vi "Measurement Logic.vi"() -> ()   [LabVIEW 2021, in "Ramp-Up Time_PMIC.lvlib"]
uses:
  Ramp-Up Time_PMIC.lvlib
  <vilib>/Plug-In SDKs/Measurements/Measure Call Context/Measure Call Context.lvclass
  Measurement Results.ctl
  Measurement Configuration.ctl
  <instrlib>/niDCPower/nidcpower.llb/niDCPower Source Mode.ctl
  <instrlib>/niDCPower/nidcpower.llb/niDCPower Wait For Event - Event.ctl
  <instrlib>/niScope/Controls/niScope trigger slope.ctl
  <instrlib>/niDCPower/nidcpower.llb/niDCPower Output Function.ctl
  <instrlib>/niDCPower/nidcpower.llb/niDCPower Aperture Time Units.ctl
  <instrlib>/niDCPower/nidcpower.llb/niDCPower Get Channel Name From String.vi
  <instrlib>/niScope/Utility/niScope Get Channel Name From String.vi
  <instrlib>/niScope/Configure/Trigger/niScope Configure Trigger Digital.vi
  <instrlib>/niDCPower/nidcpower.llb/niDCPower Configure Digital Edge Measure Trigger With Channels.vi
  <instrlib>/niDCPower/nidcpower.llb/niDCPower Configure Digital Edge Source Trigger With Channels.vi
  <instrlib>/niScope/Acquire/Fetch/niScope Fetch WDT.vi
panel:
  in  "measurement configuration":T1={"Source resource name"="", "Source current limit"=0.25, "Source sample rate"=1800000.0, "Source voltage set point 1(V1)"=7.0, "Source voltage set point 2(V2)"=20.0, "Source transient response"=1042, "Source voltage gain bandwidth"=2000.0, "Source voltage compensation frequency"=3530.0, "Source voltage pole-zero ratio"=2.0, "Source maximum power"=300.0, "Source voltage ramp rate"=6550.0, "Source voltatge V2 time"=0.005, "Source voltage V1 time"=0.005, "Load enable/disable"=TRUE, "Load resource name"="", "Load sense"=1009, "Load voltage limit range"=6.0, "Load current level"=1.0, "Scope enable/disable"=TRUE, "Scope resource name"="", "Scope output channel name"="0", "Scope sample rate"=1800000.0, "Scope probe attenuation"=1.0, "Scope vertical range"=10.0, "Scope vertical coupling"=enum."DC", "Load current level range"=4.0, "Load source delay"=1.0, "Source ramp start percentage(%)"=10.0, "Source ramp stop percentage(%)"=90.0, "Source sense"=1009} {"Source sense" items=["Local"=1008, "Remote"=1009]; "Scope vertical range" format="%.2f"; "Scope probe attenuation" format="%.1f"; "Scope sample rate" step=1000000.0 format="%#.2g"; "Load current level" format="%.1f"; "Load voltage limit range" step=1000000.0 format="%#.2g"; "Load sense" items=["Local"=1008, "Remote"=1009]; "Source voltage V1 time" format="%#_8g"; "Source transient response" items=["Slow"=1041, "Normal"=1038, "Fast"=1039, "Custom"=1042]}
  out "measurement results":T2
  out "measure call context out":refnum<class "Measure Call Context.lvclass">
  in  "measure call context in":refnum<class "Measure Call Context.lvclass">
  out "error out":errorcluster
  in  "error in":errorcluster
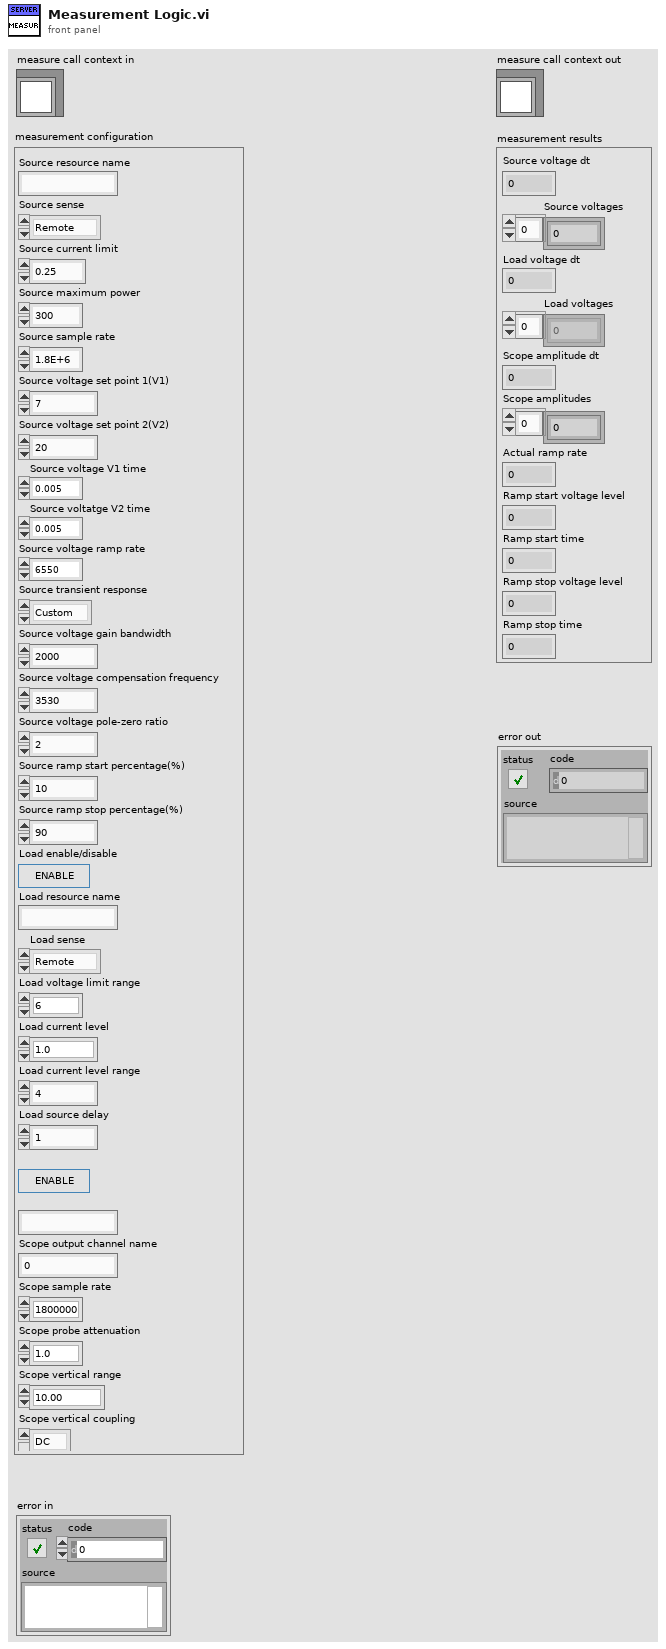
[diagram p1: front panel]
types:
  T1 = typedef "Ramp-Up Time_PMIC.lvlib/Measurement Configuration.ctl" = cluster{"Source resource name":string, "Source current limit":dbl, "Source sample rate":dbl, "Source voltage set point 1(V1)":dbl, "Source voltage set point 2(V2)":dbl, "Source transient response":i32, "Source voltage gain bandwidth":dbl, "Source voltage compensation frequency":dbl, "Source voltage pole-zero ratio":dbl, "Source maximum power":dbl, "Source voltage ramp rate":dbl, "Source voltatge V2 time":dbl, "Source voltage V1 time":dbl, "Load enable/disable":bool, "Load resource name":string, "Load sense":i32, "Load voltage limit range":dbl, "Load current level":dbl, "Scope enable/disable":bool, "Scope resource name":string, "Scope output channel name":string, "Scope sample rate":dbl, "Scope probe attenuation":dbl, "Scope vertical range":dbl, "Scope vertical coupling":enum32{"AC", "DC"}, "Load current level range":dbl, "Load source delay":dbl, "Source ramp start percentage(%)":dbl, "Source ramp stop percentage(%)":dbl, "Source sense":i32}
  T2 = typedef "Ramp-Up Time_PMIC.lvlib/Measurement Results.ctl" = cluster{"Source voltage dt":dbl, "Source voltages":dbl[], "Load voltage dt":dbl, "Load voltages":dbl[], "Scope amplitude dt":dbl, "Scope amplitudes":dbl[], "Actual ramp rate":dbl, "Ramp start voltage level":dbl, "Ramp start time":dbl, "Ramp stop voltage level":dbl, "Ramp stop time":dbl}
  T3 = cluster{"Source out":refnum<k15>, "Source channel name":string, "Load out":refnum<k15>, "Load channel name":string, "Scope out":refnum<k15>, "Scope channel name":string, "Source terminal name":string, "Start source terminal name":string, "Measure load and scope terminal name":string, "Measure record length smu":i32, "Aperture time":dbl, "Measure record length scope":i32, "measurement results":T2}
  T4 = typedef "niDCPower Wait For Event - Event.ctl" = i32
  T5 = typedef "niDCPower Source Mode.ctl" = i32
  T6 = typedef "niScope trigger slope.ctl" = i32
  T7 = typedef "niDCPower Aperture Time Units.ctl" = i32
  T8 = typedef "niDCPower Output Function.ctl" = i32
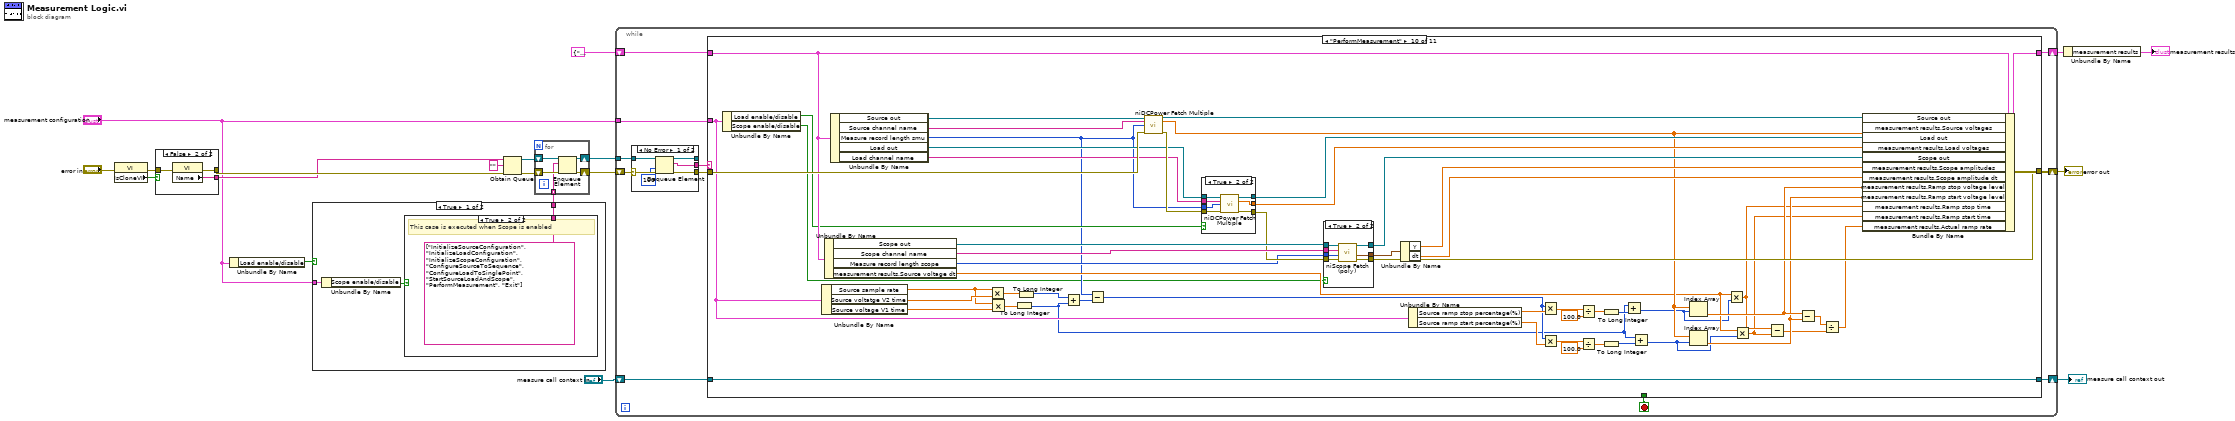
[diagram p0: block diagram]
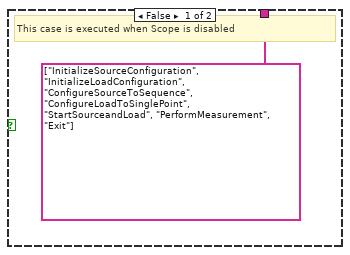
[diagram p2: hidden frame]
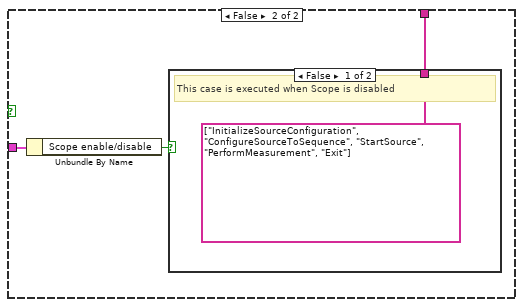
[diagram p3: hidden frame]
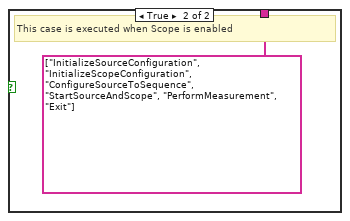
[diagram p4: hidden frame]
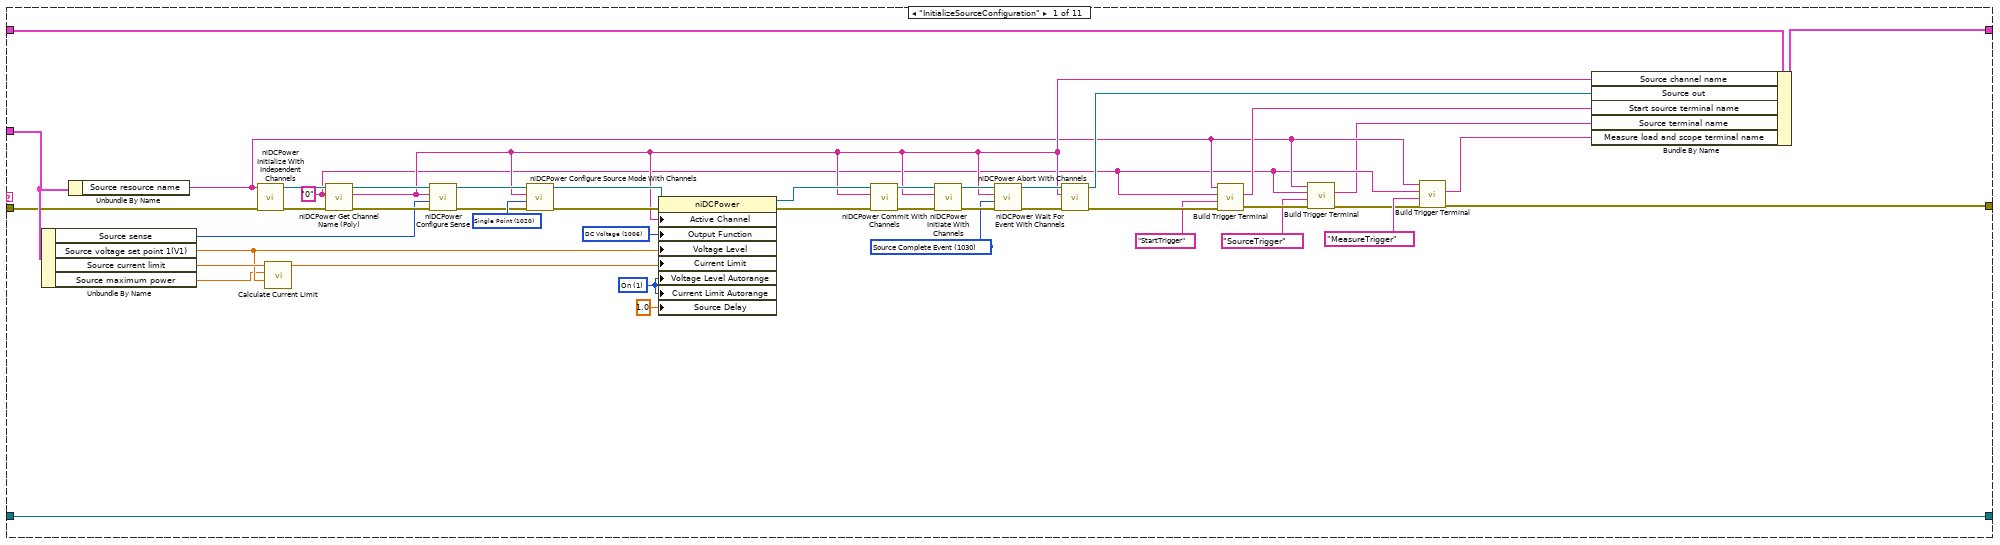
[diagram p5: hidden frame]
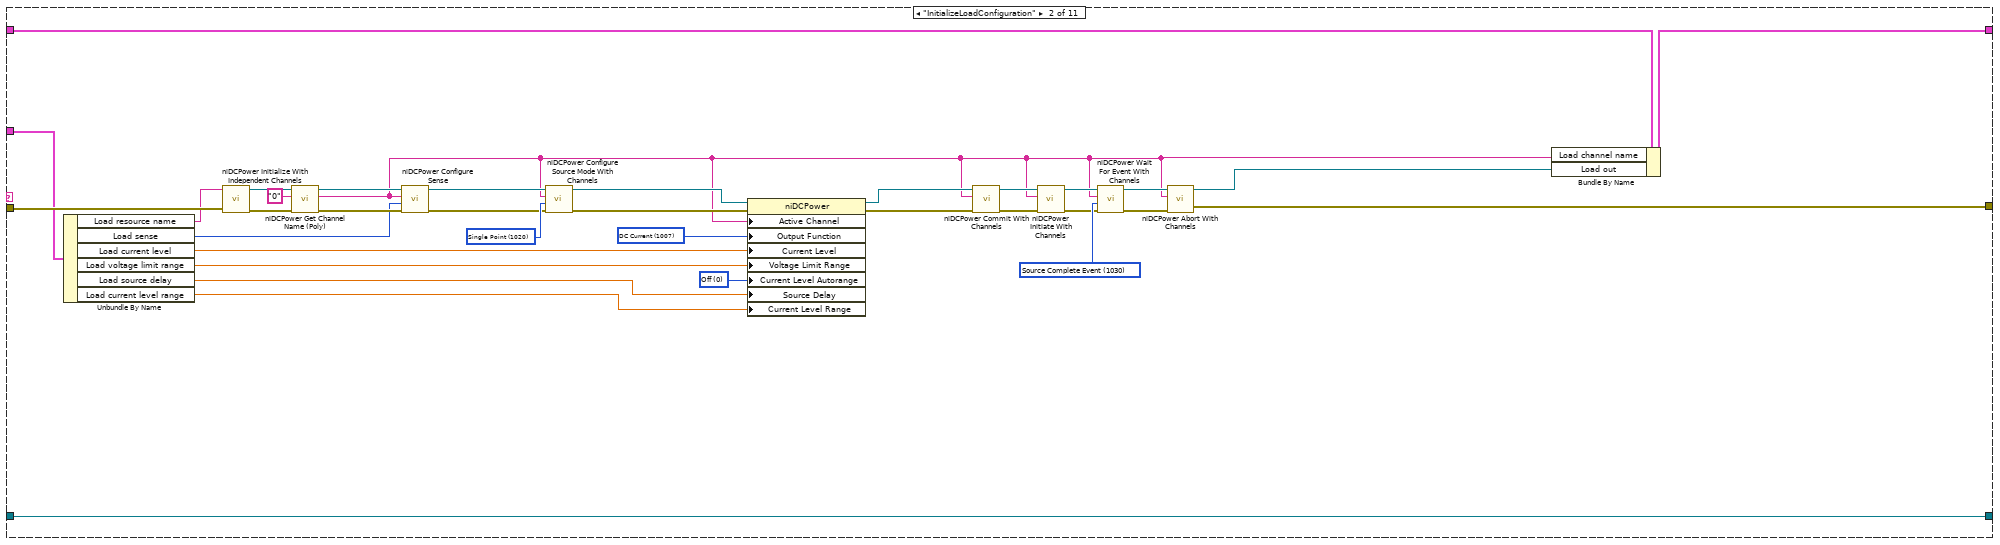
[diagram p6: hidden frame]
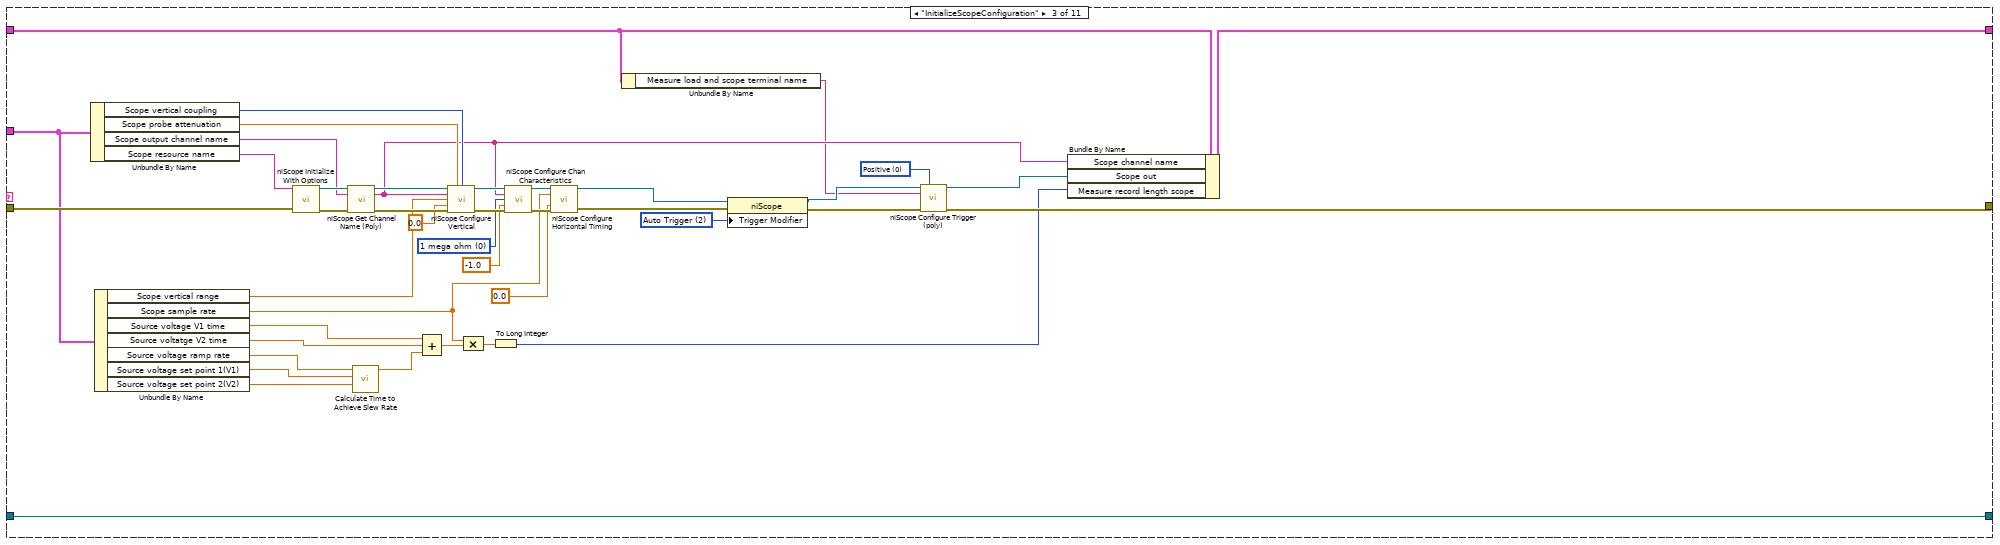
[diagram p7: hidden frame]
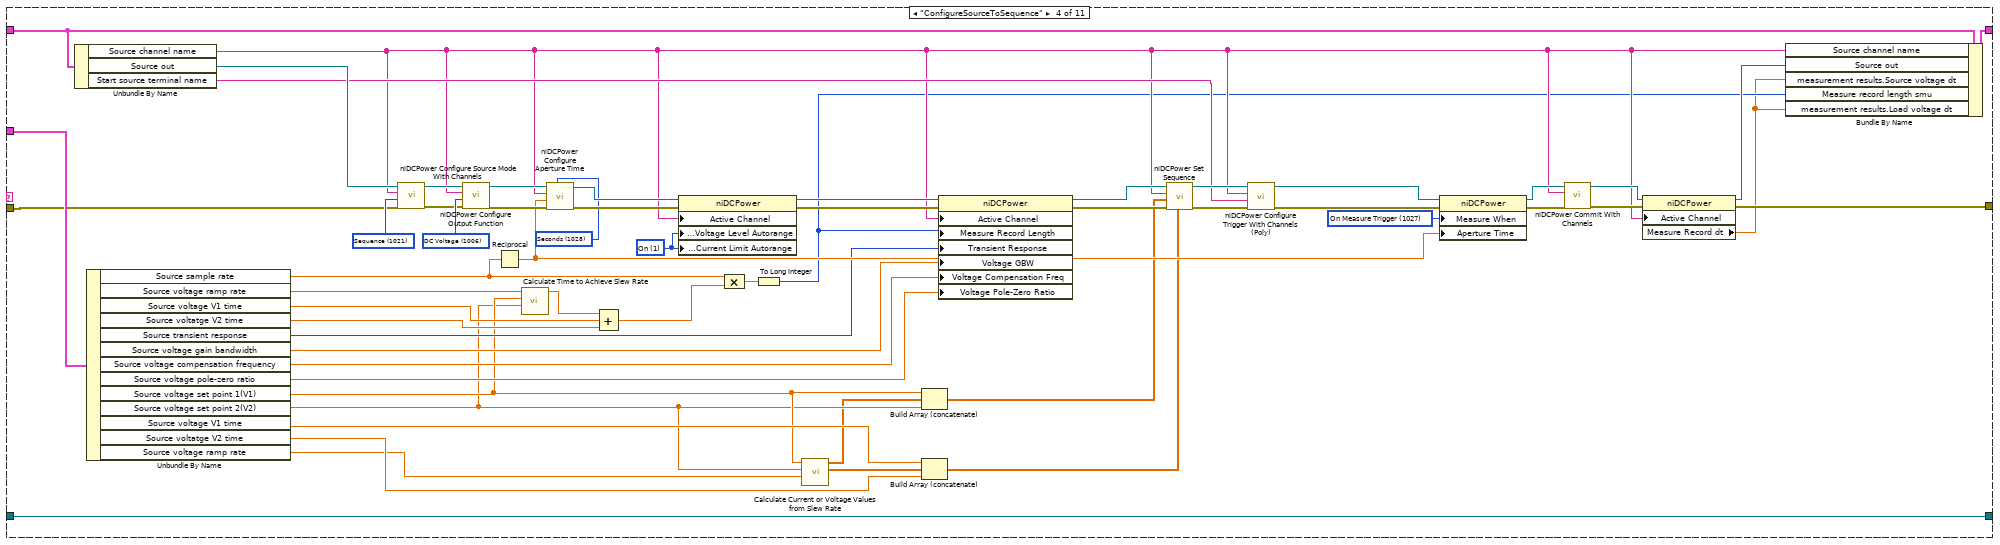
[diagram p8: hidden frame]
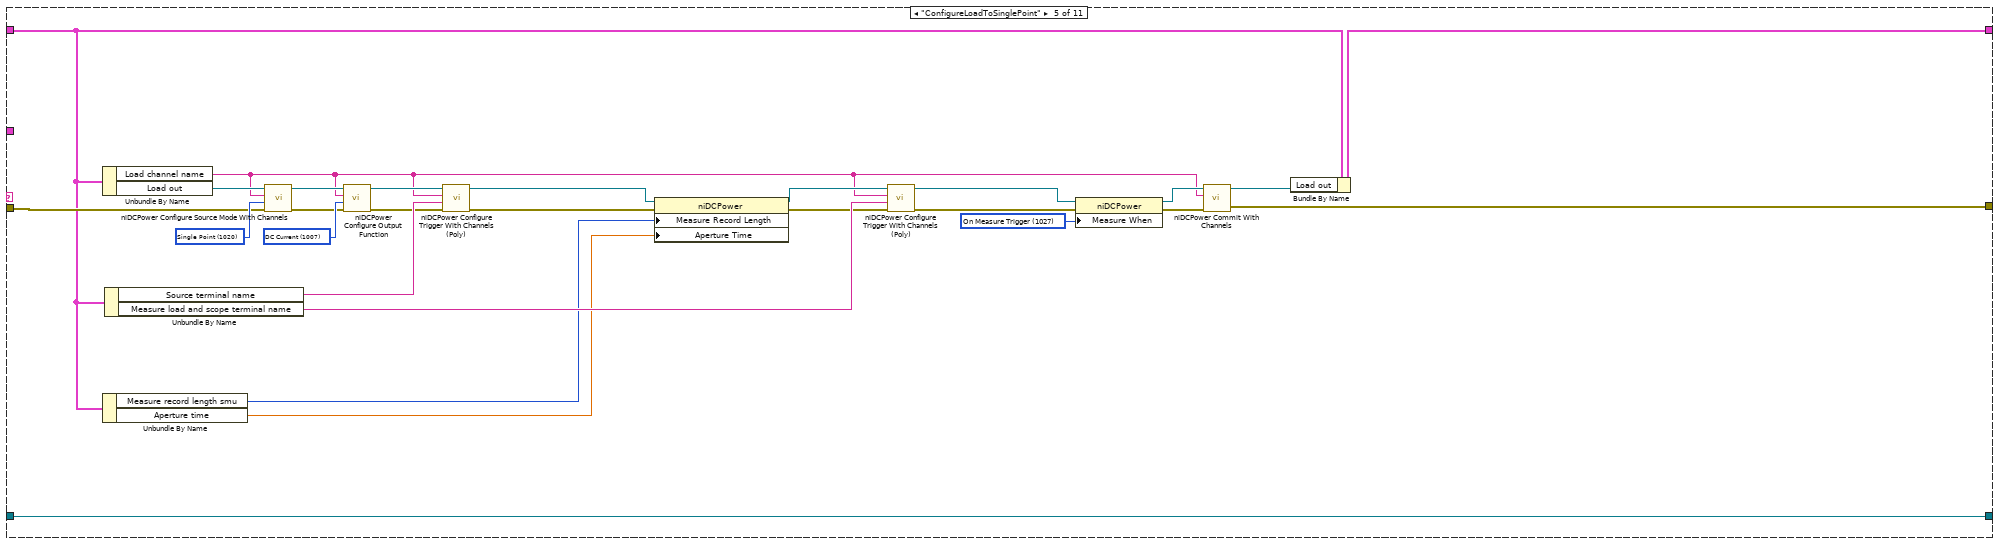
[diagram p9: hidden frame]
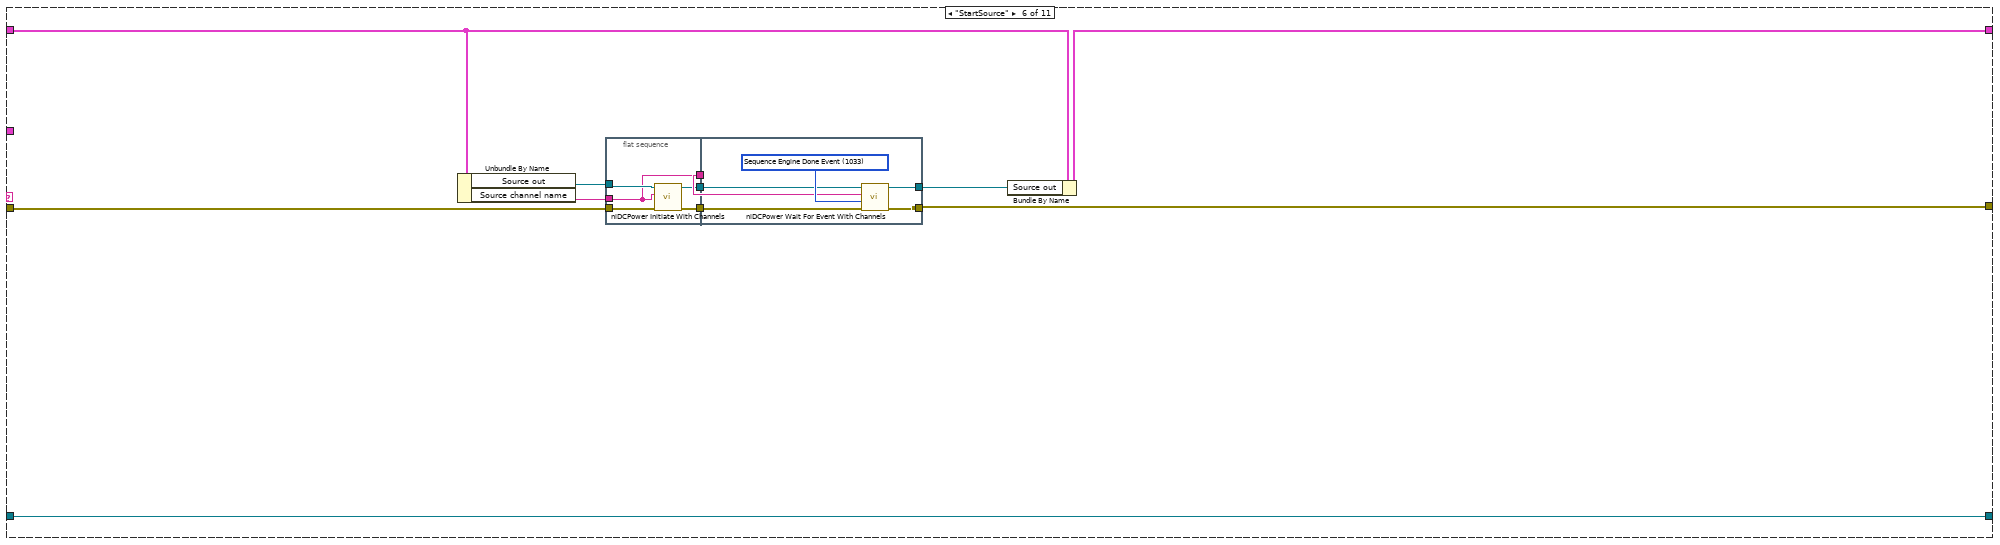
[diagram p10: hidden frame]
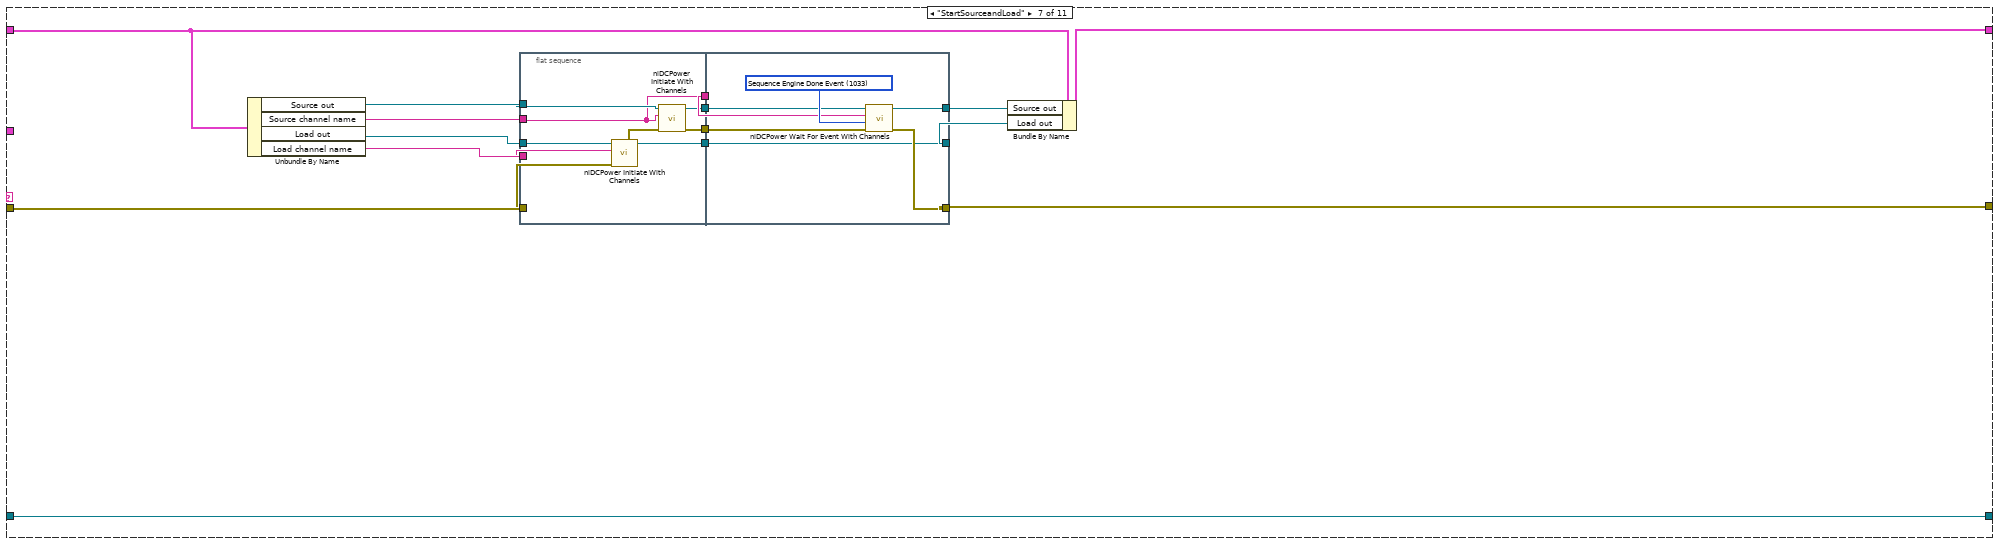
[diagram p11: hidden frame]
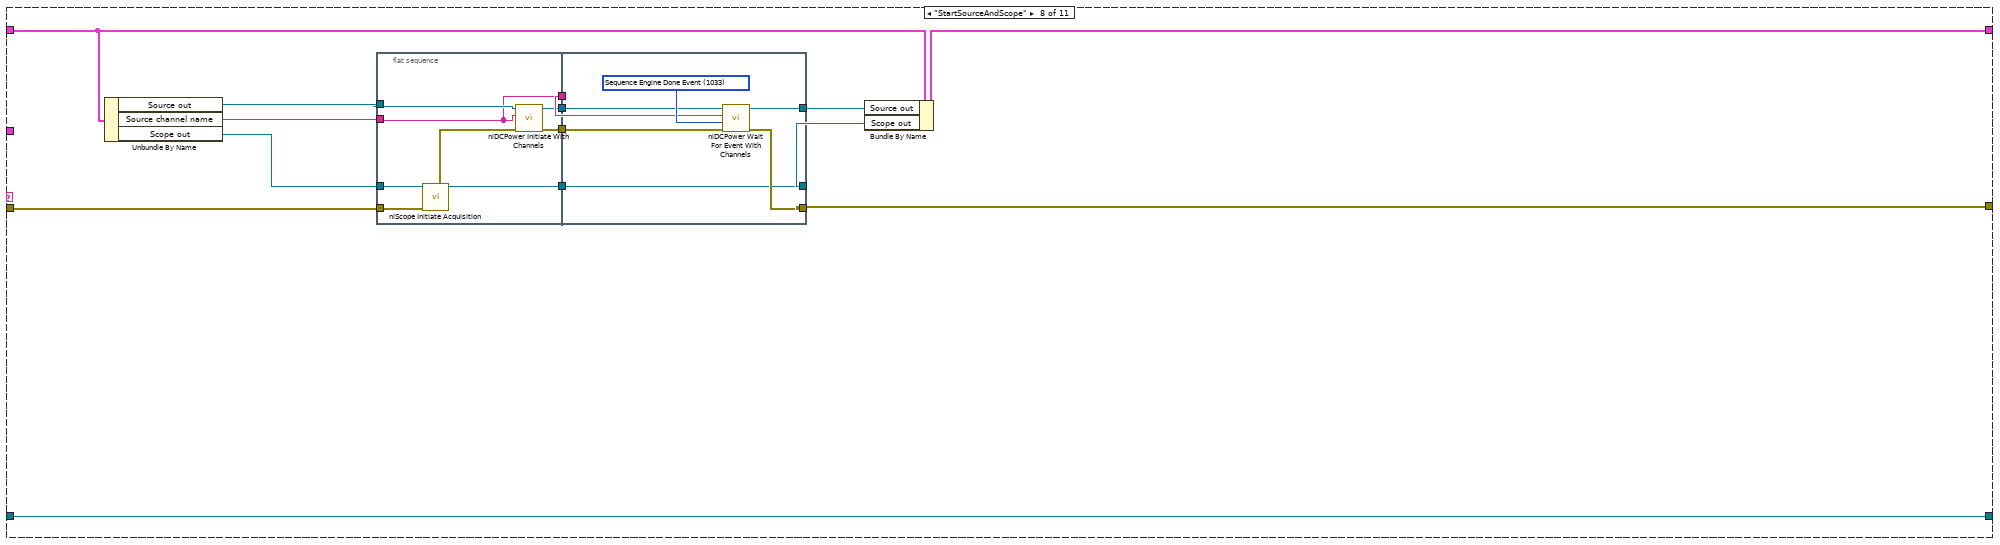
[diagram p12: hidden frame]
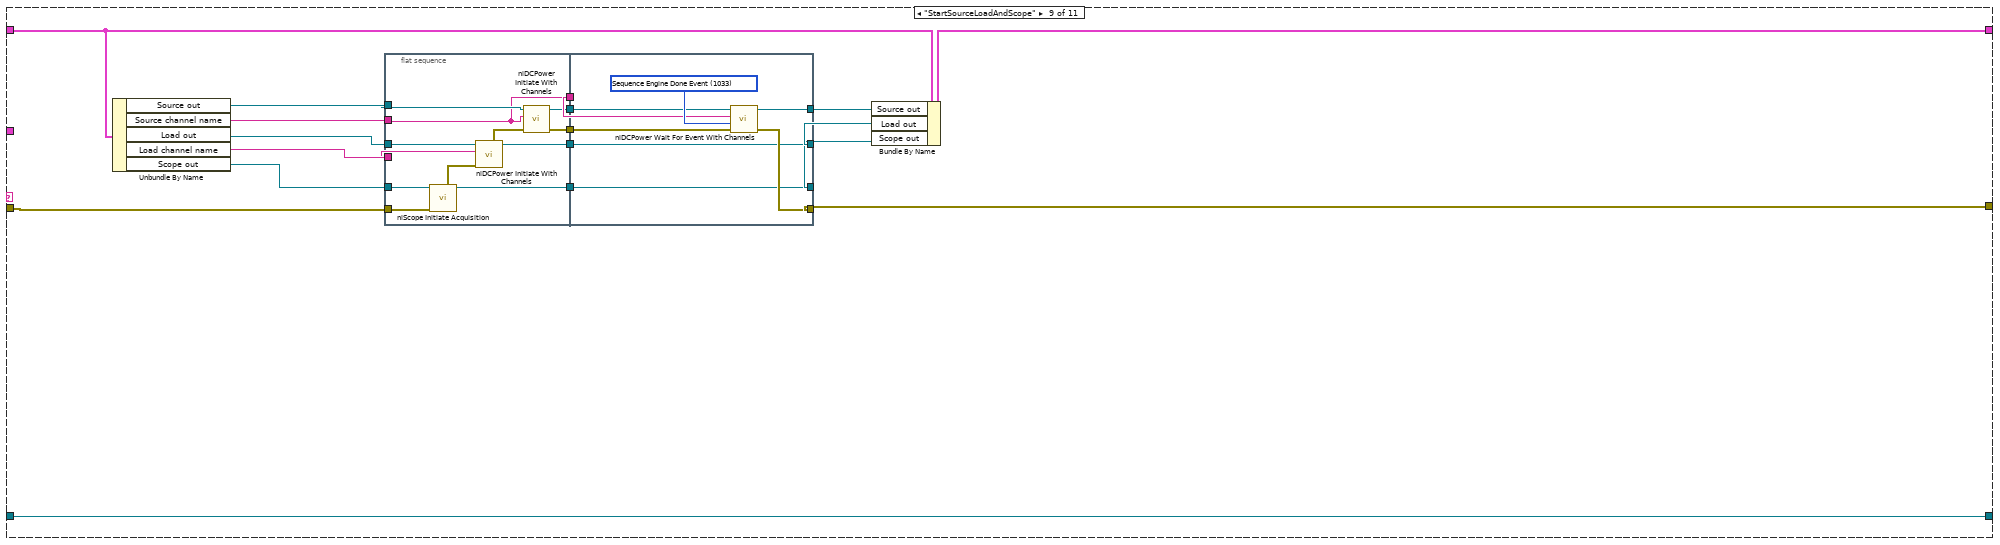
[diagram p13: hidden frame]
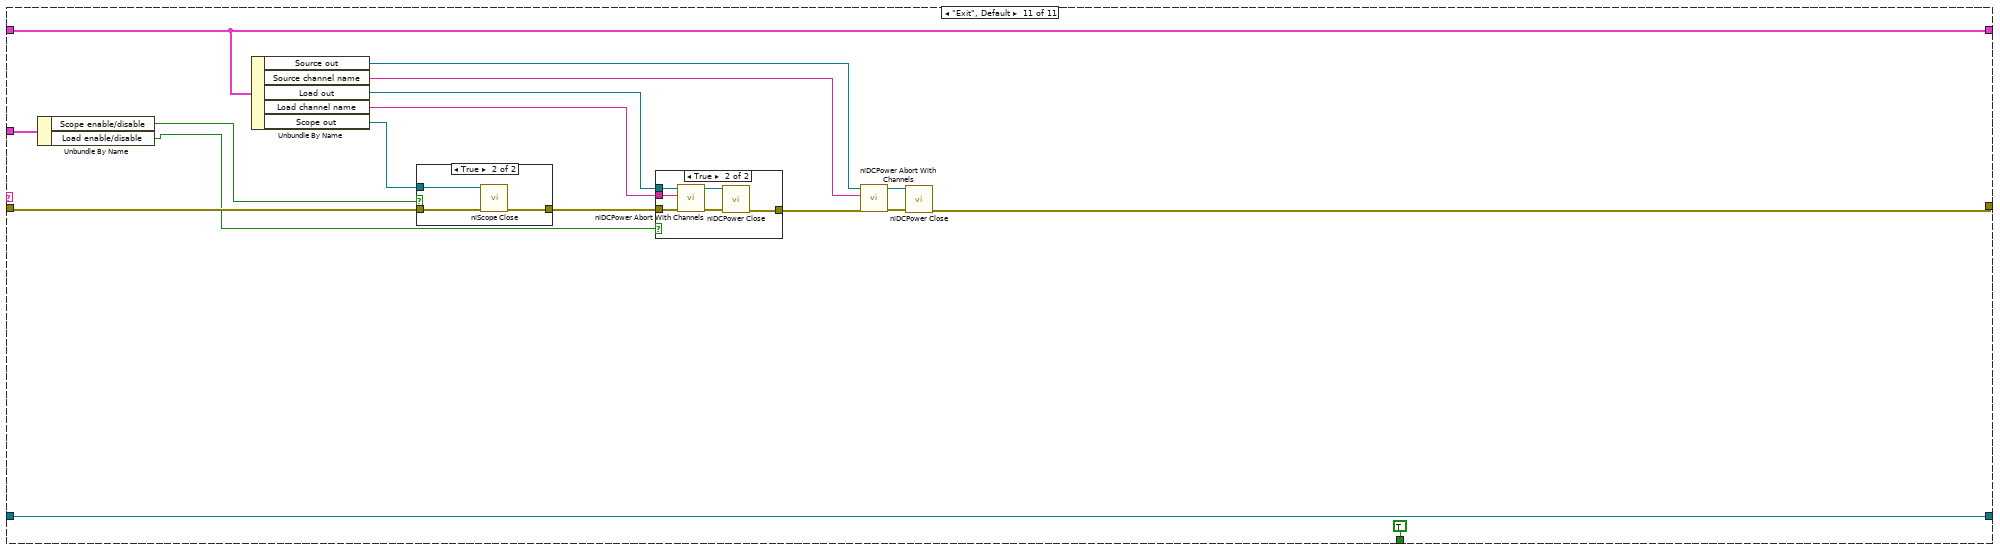
[diagram p16: hidden frame]
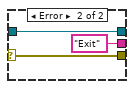
[diagram p19: hidden frame]
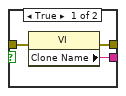
[diagram p20: hidden frame]
diagram:
  n1 = property class="VI"(error in="error in") -> (error out=w18:errorcluster, "IsCloneVI"=w19:bool)  [unwired: 1 in, 1 out]
  n2 = case shown="False" w19 {
    tunnel: [w22 w25] -> w17
    tunnel: [w21 w24] -> w16
    tunnel: w18 -> [w20 w23]
    frame True {
      n3 = property class="VI"(error in=w20) -> (error out=w22:errorcluster, "Clone Name"=w21:string)  [unwired: 1 in, 1 out]
    }
    frame False {
      n4 = property class="VI"(error in=w23) -> (error out=w25:errorcluster, "Name"=w24:string)  [unwired: 1 in, 1 out]
    }
  }
  n5 = Unbundle By Name("measurement configuration") -> ("Load enable/disable"=w3:bool)
  n6 = case shown="True" w3 {
    tunnel: [w26 w33] -> w12
    tunnel: "measurement configuration" -> [w27 w31]
    frame True {
      n7 = Unbundle By Name(w27) -> ("Scope enable/disable"=w28:bool)
      n8 = case shown="True" w28 {
        tunnel: [string[] ["InitializeSourceConfiguration", "InitializeLoadConfiguration", "ConfigureSourceToSequence", "ConfigureLoadToSinglePoint", "StartSourceandLoad", "PerformMeasurement", "Exit"] ("Step sequence") string[] ["InitializeSourceConfiguration", "InitializeLoadConfiguration", "InitializeScopeConfiguration", "ConfigureSourceToSequence", "ConfigureLoadToSinglePoint", "StartSourceLoadAndScope", "PerformMeasurement", "Exit"] ("Step sequence")] -> w26
        frame False {
          # "This case is executed when Scope is disabled"
        }
        frame True {
          # "This case is executed when Scope is enabled"
        }
      }
    }
    frame False {
      n9 = Unbundle By Name(w31) -> ("Scope enable/disable"=w32:bool)
      n10 = case shown="False" w32 {
        tunnel: [string[] ["InitializeSourceConfiguration", "ConfigureSourceToSequence", "StartSource", "PerformMeasurement", "Exit"] ("Step sequence") string[] ["InitializeSourceConfiguration", "InitializeScopeConfiguration", "ConfigureSourceToSequence", "StartSourceAndScope", "PerformMeasurement", "Exit"] ("Step sequence")] -> w33
        frame False {
          # "This case is executed when Scope is disabled"
        }
        frame True {
          # "This case is executed when Scope is enabled"
        }
      }
    }
  }
  n11 = Obtain Queue(name (unnamed)=w16, element data type="", error in (no error)=w17) -> (queue out=w14:refnum<queue>, error out=w15:errorcluster)  [unwired: 2 in, 1 out]
  n12 = for {
    shift-right: [w38] -> w11
    shift-left: w14 -> [w40]
    shift-right: [w37] -> w10
    shift-left: w15 -> [w39]
    tunnel: w12 -> [w36] mode=indexing
    n13 = Enqueue Element(queue=w40, element=w36, error in (no error)=w39) -> (queue out=w38:refnum<queue>, error out=w37:errorcluster)  [unwired: 1 in, 1 out]
  }
  n14 = while {
    tunnel: w11 -> [w51]
    shift-right: [w44] -> w8
    shift-left: w10 -> [w50]
    tunnel: "measurement configuration" -> [w48]
    shift-right: [w46] -> w6
    shift-left: T3 {"Source out"="", "Source channel name"="", "Load out"="", "Load channel name"="", "Scope out"="", "Scope channel name"="", "Source terminal name"="", "Start source terminal name"="", "Measure load and scope terminal name"="", "Measure record length smu"=0, "Aperture time"=0.0, "Measure record length scope"=0, "measurement results"={"Source voltage dt"=0.0, "Source voltages"=[0.0], "Load voltage dt"=0.0, "Load voltages"=[], "Scope amplitude dt"=0.0, "Scope amplitudes"=[0.0], "Actual ramp rate"=0.0, "Ramp start voltage level"=0.0, "Ramp start time"=0.0, "Ramp stop voltage level"=0.0, "Ramp stop time"=0.0}} -> [w47]
    shift-right: [w42] -> w1
    shift-left: "measure call context in" -> [w41]
    stop <- w43 stop-if-true
    n15 = case shown="No Error" w50 {
      selector: w50 -> [w481 w485]
      tunnel: w51 -> [w483 w484]
      tunnel: [w482 "Exit" ("t")] -> w49
      tunnel: [w480 w485] -> w45
      tunnel: [w478 w484] -> _
      frame No Error {
        n16 = Dequeue Element(queue=w483, timeout in ms (-1)=100, error in (no error)=w481) -> (queue out=w478:refnum<queue>, element=w482:string, error out=w480:errorcluster)  [unwired: 1 out]
      }
      frame Error {
      }
    }
    n17 = case shown="\"PerformMeasurement\"" w49 {
      tunnel: w48 -> [w74 w102 w143 w195 _ _ _ _ _ w392 w462]
      tunnel: w47 -> [w73 w99 w140 w194 w232 w261 w281 w317 w341 w430 w463]
      tunnel: [w72 w100 w173 w229 w231 w260 w280 w312 w340 w429 w463] -> w46
      tunnel: w45 -> [w71 w103 w144 w192 w233 w262 w282 w316 w342 w431 w466]
      tunnel: [w57 w101 w138 w183 w230 w259 w279 w313 w339 w428 w465] -> w44
      tunnel: [_ _ _ _ _ _ _ _ _ _ TRUE] -> w43
      tunnel: [w69 w131 w137 w188 w256 w258 w293 w311 w356 w421 w456] -> w42
      tunnel: w41 -> [w69 w131 w137 w188 w256 w258 w293 w311 w356 w421 w456]
      frame "InitializeSourceConfiguration" {
        w55 = "0" ("index")
        w80 = 1 items=["Off", "On"] ("Source:DC Voltage:Voltage Level Autorange")
        w81 = T4 1030 items=["Source Complete Event"=1030, "Measure Complete Event"=1031, "Sequence Iteration Complete Event"=1032, "Sequence Engine Done Event"=1033, "Pulse Complete Event"=1051, "Ready For Pulse Trigger Event"=1052] ("event")
        w92 = T5 1020 items=["Single Point"=1020, "Sequence"=1021] ("source mode")
        w87 = 1006 items=["DC Voltage"=1006, "DC Current"=1007, "Pulse Voltage"=1049, "Pulse Current"=1050] ("Source:Output Function")
        n18 = Unbundle By Name(w74) -> ("Source sense"=w52:i32, "Source voltage set point 1(V1)"=w67:dbl, "Source current limit"=w68:dbl, "Source maximum power"=w66:dbl)
        n19 = Unbundle By Name(w74) -> ("Source resource name"=w56:string)
        n20 = call <instrlib>:"niDCPower Initialize With Independent Channels.vi"("error in (no error)"=w71, "resource name"=w56) -> ("error out"=w78:errorcluster, "instrument handle out"=w82:refnum<k15>)  [unwired: 8 in]
        n21 = call "Calculate Current Limit.vi"("Voltage value"=w67, "Maximum power"=w66, "Current limit in"=w68) -> ("Current limit out"=w65:dbl)  [unwired: 8 in]
        n22 = call-poly <instrlib>:"niDCPower Get Channel Name (Poly).vi"("error in (no error)"=w78, "index"=w55, "instrument handle"=w82) -> ("error out"=w77:errorcluster, "name"=w76:string, "instrument handle out"=w79:refnum<k15>)  [unwired: 6 in]
        n23 = call <instrlib>:"niDCPower Configure Sense.vi"("error in (no error)"=w77, "sense"=w52, "channel name"=w76, "instrument handle"=w79) -> ("error out"=w90:errorcluster, "instrument handle out"=w88:refnum<k15>)  [unwired: 6 in]
        n24 = call <instrlib>:"niDCPower Configure Source Mode With Channels.vi"("error in (no error)"=w90, "source mode"=w92, "channel name"=w76, "instrument handle"=w88) -> ("error out"=w91:errorcluster, "instrument handle out"=w89:refnum<k15>)  [unwired: 6 in]
        n25 = property class="niDCPower"(reference=w89, error in=w91, "Active Channel"=w76, "Output Function"=w87, "Voltage Level"=w67, "Current Limit"=w65, "Voltage Level Autorange"=w80, "Current Limit Autorange"=w80, "Source Delay"=1.0 ("Source:Advanced:Source Delay")) -> (reference out=w93:refnum<k15>, error out=w94:errorcluster)
        n26 = call <instrlib>:"niDCPower Commit With Channels.vi"("error in (no error)"=w94, "channel name"=w76, "instrument handle"=w93) -> ("error out"=w96:errorcluster, "instrument handle out"=w95:refnum<k15>)  [unwired: 7 in]
        n27 = call <instrlib>:"niDCPower Initiate With Channels.vi"("error in (no error)"=w96, "channel name"=w76, "instrument handle"=w95) -> ("error out"=w83:errorcluster, "instrument handle out"=w84:refnum<k15>)  [unwired: 7 in]
        n28 = call <instrlib>:"niDCPower Wait For Event With Channels.vi"("error in (no error)"=w83, "event"=w81, "channel name"=w76, "instrument handle"=w84) -> ("error out"=w86:errorcluster, "instrument handle out"=w85:refnum<k15>)  [unwired: 6 in]
        n29 = call <instrlib>:"niDCPower Abort With Channels.vi"("error in (no error)"=w86, "channel name"=w76, "instrument handle"=w85) -> ("error out"=w64:errorcluster, "instrument handle out"=w75:refnum<k15>)  [unwired: 7 in]
        n30 = call "Build Trigger Terminal.vi"("error in (no error)"=w64, "Trigger/Event Name"="StartTrigger", "Channel Name"=w55, "Resource Name"=w56) -> ("error out"=w62:errorcluster, "Terminal Name"=w60:string)  [unwired: 6 in]
        n31 = call "Build Trigger Terminal.vi"("error in (no error)"=w62, "Trigger/Event Name"="SourceTrigger", "Channel Name"=w55, "Resource Name"=w56) -> ("error out"=w58:errorcluster, "Terminal Name"=w53:string)  [unwired: 6 in]
        n32 = call "Build Trigger Terminal.vi"("error in (no error)"=w58, "Trigger/Event Name"="MeasureTrigger", "Channel Name"=w55, "Resource Name"=w56) -> ("error out"=w57:errorcluster, "Terminal Name"=w54:string)  [unwired: 6 in]
        n33 = Bundle By Name(cluster=w73, "Source channel name"=w76, "Source out"=w75, "Start source terminal name"=w60, "Source terminal name"=w53, "Measure load and scope terminal name"=w54) -> (w72:T3)
      }
      frame "InitializeLoadConfiguration" {
        w126 = T5 1020 items=["Single Point"=1020, "Sequence"=1021] ("source mode")
        w119 = T4 1030 items=["Source Complete Event"=1030, "Measure Complete Event"=1031, "Sequence Iteration Complete Event"=1032, "Sequence Engine Done Event"=1033, "Pulse Complete Event"=1051, "Ready For Pulse Trigger Event"=1052] ("event")
        w114 = 0 items=["Off", "On"] ("Source:DC Current:Current Level Autorange")
        w115 = 1007 items=["DC Voltage"=1006, "DC Current"=1007, "Pulse Voltage"=1049, "Pulse Current"=1050] ("Source:Output Function")
        n34 = Unbundle By Name(w102) -> ("Load resource name"=w98:string, "Load sense"=w97:i32, "Load current level"=w108:dbl, "Load voltage limit range"=w107:dbl, "Load source delay"=w113:dbl, "Load current level range"=w106:dbl)
        n35 = call <instrlib>:"niDCPower Initialize With Independent Channels.vi"("error in (no error)"=w103, "resource name"=w98) -> ("error out"=w111:errorcluster, "instrument handle out"=w116:refnum<k15>)  [unwired: 8 in]
        n36 = call-poly <instrlib>:"niDCPower Get Channel Name (Poly).vi"("error in (no error)"=w111, "index"="0", "instrument handle"=w116) -> ("error out"=w110:errorcluster, "name"=w104:string, "instrument handle out"=w112:refnum<k15>)  [unwired: 6 in]
        n37 = call <instrlib>:"niDCPower Configure Sense.vi"("error in (no error)"=w110, "sense"=w97, "channel name"=w104, "instrument handle"=w112) -> ("error out"=w123:errorcluster, "instrument handle out"=w122:refnum<k15>)  [unwired: 6 in]
        n38 = call <instrlib>:"niDCPower Configure Source Mode With Channels.vi"("error in (no error)"=w123, "source mode"=w126, "channel name"=w104, "instrument handle"=w122) -> ("error out"=w125:errorcluster, "instrument handle out"=w124:refnum<k15>)  [unwired: 6 in]
        n39 = property class="niDCPower"(reference=w124, error in=w125, "Active Channel"=w104, "Output Function"=w115, "Current Level"=w108, "Voltage Limit Range"=w107, "Current Level Autorange"=w114, "Source Delay"=w113, "Current Level Range"=w106) -> (reference out=w127:refnum<k15>, error out=w128:errorcluster)
        n40 = call <instrlib>:"niDCPower Commit With Channels.vi"("error in (no error)"=w128, "channel name"=w104, "instrument handle"=w127) -> ("error out"=w129:errorcluster, "instrument handle out"=w130:refnum<k15>)  [unwired: 7 in]
        n41 = call <instrlib>:"niDCPower Initiate With Channels.vi"("error in (no error)"=w129, "channel name"=w104, "instrument handle"=w130) -> ("error out"=w117:errorcluster, "instrument handle out"=w118:refnum<k15>)  [unwired: 7 in]
        n42 = call <instrlib>:"niDCPower Wait For Event With Channels.vi"("error in (no error)"=w117, "event"=w119, "channel name"=w104, "instrument handle"=w118) -> ("error out"=w121:errorcluster, "instrument handle out"=w120:refnum<k15>)  [unwired: 6 in]
        n43 = call <instrlib>:"niDCPower Abort With Channels.vi"("error in (no error)"=w121, "channel name"=w104, "instrument handle"=w120) -> ("error out"=w101:errorcluster, "instrument handle out"=w109:refnum<k15>)  [unwired: 7 in]
        n44 = Bundle By Name(cluster=w99, "Load channel name"=w104, "Load out"=w109) -> (w100:T3)
      }
      frame "InitializeScopeConfiguration" {
        w161 = 2 items=["None"=1, "Auto Trigger"=2] ("Trigger Modifier")
        w152 = u32 0 items=["1 mega ohm"=0, "50 ohms"=2] ("Input Impedance")
        w158 = T6 0 items=["Positive", "Negative"] ("trigger slope")
        n45 = Unbundle By Name(w143) -> ("Scope vertical coupling"=w155:enum32{"AC", "DC"}, "Scope probe attenuation"=w156:dbl, "Scope output channel name"=w153:string, "Scope resource name"=w157:string)
        n46 = Unbundle By Name(w143) -> ("Scope vertical range"=w151:dbl, "Scope sample rate"=w154:dbl, "Source voltage V1 time"=w149:dbl, "Source voltatge V2 time"=w148:dbl, "Source voltage ramp rate"=w135:dbl, "Source voltage set point 1(V1)"=w134:dbl, "Source voltage set point 2(V2)"=w133:dbl)
        n47 = call <instrlib>:"niScope Initialize With Options.vi"("resource name"=w157, "error in"=w144) -> ("instrument handle"=w172:refnum<k15>, "error out"=w171:errorcluster)  [unwired: 12 in]
        n48 = call-poly <instrlib>:"niScope Get Channel Name (Poly).vi"("instrument handle"=w172, "index"=w153, "error in"=w171) -> ("instrument handle out"=w160:refnum<k15>, "channel name"=w141:string, "error out"=w159:errorcluster)  [unwired: 10 in]
        n49 = call "Calculate Time to Achieve Slew Rate.vi"("Current/voltage set point 2"=w133, "Current/voltage set point 1"=w134, "Current/voltage slew rate"=w135) -> ("Calculated time"=w136:dbl)  [unwired: 8 in]
        n50 = Compound Arithmetic op=ADD(w149, w148, w136) -> (w145:dbl)
        n51 = call <instrlib>:"niScope Configure Vertical.vi"("instrument handle"=w160, "probe attenuation"=w156, "vertical coupling"=w155, "channels"=w141, "vertical range"=w151, "vertical offset"=0.0, "error in"=w159) -> ("instrument handle out"=w170:refnum<k15>, "error out"=w169:errorcluster)  [unwired: 7 in]
        n52 = Compound Arithmetic op=MULTIPLY(w154, w145) -> (w146:dbl)
        n53 = To Long Integer(number=w146) -> (32bit integer=w132:i32)
        n54 = call <instrlib>:"niScope Configure Chan Characteristics.vi"("instrument handle"=w170, "channels"=w141, "input impedance"=w152, "maximum input frequency"=-1.0 ("Maximum Input Frequency"), "error in"=w169) -> ("instrument handle out"=w167:refnum<k15>, "error out"=w168:errorcluster)  [unwired: 9 in]
        n55 = call <instrlib>:"niScope Configure Horizontal Timing.vi"("instrument handle"=w167, "min sample rate"=w154, "reference position"=0.0 ("Reference Position"), "error in"=w168) -> ("instrument handle out"=w164:refnum<k15>, "error out"=w163:errorcluster)  [unwired: 10 in]
        n56 = Unbundle By Name(w140) -> ("Measure load and scope terminal name"=w139:string)
        n57 = property on="Property Node" class="niScope"(reference=w164, error in=w163, "Trigger Modifier"=w161) -> (reference out=w147:refnum<k15>, error out=w162:errorcluster)
        n58 = call-poly <instrlib>:"niScope Configure Trigger (poly).vi"("instrument handle"=w147, "trigger slope"=w158, "trigger source"=w139, "error in"=w162) -> ("instrument handle out"=w142:refnum<k15>, "error out"=w138:errorcluster)  [unwired: 10 in]
        n59 = Bundle By Name(cluster=w140, "Scope channel name"=w141, "Scope out"=w142, "Measure record length scope"=w132) -> (w173:T3)
      }
      frame "ConfigureSourceToSequence" {
        w214 = T7 1028 items=["Seconds"=1028, "Powerline Cycles"=1029] ("aperture time units")
        w221 = 1027 items=["Automatically after Source Complete"=1025, "On Demand"=1026, "On Measure Trigger"=1027] ("Measurement:Advanced:Measure When")
        w226 = 1 items=["Off", "On"] ("DC Voltage:Voltage Level Autorange")
        w225 = T8 1006 items=["DC Voltage"=1006, "DC Current"=1007, "Pulse Voltage"=1049, "Pulse Current"=1050] ("output function")
        w224 = T5 1021 items=["Single Point"=1020, "Sequence"=1021] ("source mode")
        n60 = Unbundle By Name(w194) -> ("Source channel name"=w184:string, "Source out"=w193:refnum<k15>, "Start source terminal name"=w191:string)
        n61 = Unbundle By Name(w195) -> ("Source sample rate"=w201:dbl, "Source voltage ramp rate"=w181:dbl, "Source voltage V1 time"=w190:dbl, "Source voltatge V2 time"=w200:dbl, "Source transient response"=w189:i32, "Source voltage gain bandwidth"=w213:dbl, "Source voltage compensation frequency"=w212:dbl, "Source voltage pole-zero ratio"=w211:dbl, "Source voltage set point 1(V1)"=w180:dbl, "Source voltage set point 2(V2)"=w179:dbl, "Source voltage V1 time"=w199:dbl, "Source voltatge V2 time"=w198:dbl, "Source voltage ramp rate"=w178:dbl)
        n62 = call <instrlib>:"niDCPower Configure Source Mode With Channels.vi"("error in (no error)"=w192, "source mode"=w224, "channel name"=w184, "instrument handle"=w193) -> ("error out"=w222:errorcluster, "instrument handle out"=w223:refnum<k15>)  [unwired: 6 in]
        n63 = call <instrlib>:"niDCPower Configure Output Function.vi"("error in (no error)"=w222, "output function"=w225, "channel name"=w184, "instrument handle"=w223) -> ("error out"=w218:errorcluster, "instrument handle out"=w216:refnum<k15>)  [unwired: 6 out]
        n64 = Reciprocal(x=w201) -> (1/x=w206:dbl)
        n65 = call "Calculate Time to Achieve Slew Rate.vi"("Current/voltage set point 2"=w179, "Current/voltage set point 1"=w180, "Current/voltage slew rate"=w181) -> ("Calculated time"=w182:dbl)  [unwired: 8 in]
        n66 = call <instrlib>:"niDCPower Configure Aperture Time.vi"("aperture time units"=w214, "error in (no error)"=w218, "aperture time"=w206, "channel name"=w184, "instrument handle"=w216) -> ("error out"=w217:errorcluster, "instrument handle out"=w215:refnum<k15>)  [unwired: 5 in]
        n67 = Compound Arithmetic op=ADD(w182, w190, w200) -> (w207:dbl)
        n68 = property class="niDCPower"(reference=w215, error in=w217, "Active Channel"=w184, "Source:DC Voltage:Voltage Level Autorange"=w226, "Source:DC Voltage:Current Limit Autorange"=w226) -> (reference out=w227:refnum<k15>, error out=w228:errorcluster)
        n69 = Compound Arithmetic op=MULTIPLY(w201, w207) -> (w210:dbl)
        n70 = To Long Integer(number=w210) -> (32bit integer=w175:i32)
        n71 = call "Calculate Current or Voltage Values from Slew Rate.vi"("Current/voltage slew rate"=w178, "Current/voltage end point"=w179, "Current/voltage start point"=w180) -> ("Source delays"=w176:dbl[], "Current/voltage values"=w177:dbl[])  [unwired: 7 in]
        n72 = Build Array (concatenate)(w180, w177, w179) -> (w196:dbl[])
        n73 = Build Array (concatenate)(w199, w176, w198) -> (w197:dbl[])
        n74 = property class="niDCPower"(reference=w227, error in=w228, "Active Channel"=w184, "Measure Record Length"=w175, "Transient Response"=w189, "Voltage GBW"=w213, "Voltage Compensation Freq"=w212, "Voltage Pole-Zero Ratio"=w211) -> (reference out=w208:refnum<k15>, error out=w209:errorcluster)
        n75 = call <instrlib>:"niDCPower Set Sequence.vi"("source delays"=w197, "error in (no error)"=w209, "values"=w196, "channel name"=w184, "instrument handle"=w208) -> ("error out"=w204:errorcluster, "instrument handle out"=w205:refnum<k15>)  [unwired: 5 in]
        n76 = call-poly <instrlib>:"niDCPower Configure Trigger With Channels (Poly).vi"("error in (no error)"=w204, "input terminal"=w191, "channel name"=w184, "instrument handle"=w205) -> ("error out"=w202:errorcluster, "instrument handle out"=w203:refnum<k15>)  [unwired: 6 in]
        n77 = property class="niDCPower"(reference=w203, error in=w202, "Measure When"=w221, "Aperture Time"=w206) -> (reference out=w219:refnum<k15>, error out=w220:errorcluster)
        n78 = call <instrlib>:"niDCPower Commit With Channels.vi"("error in (no error)"=w220, "channel name"=w184, "instrument handle"=w219) -> ("error out"=w187:errorcluster, "instrument handle out"=w186:refnum<k15>)  [unwired: 7 in]
        n79 = property class="niDCPower"(reference=w186, error in=w187, "Active Channel"=w184) -> (reference out=w185:refnum<k15>, error out=w183:errorcluster, "Measure Record dt"=w174:dbl)
        n80 = Bundle By Name(cluster=w194, "Source channel name"=w184, "Source out"=w185, "measurement results.Source voltage dt"=w174, "Measure record length smu"=w175, "measurement results.Load voltage dt"=w174) -> (w229:T3)
      }
      frame "ConfigureLoadToSinglePoint" {
        w239 = 1027 items=["Automatically after Source Complete"=1025, "On Demand"=1026, "On Measure Trigger"=1027] ("Measurement:Advanced:Measure When")
        w249 = T8 1007 items=["DC Voltage"=1006, "DC Current"=1007, "Pulse Voltage"=1049, "Pulse Current"=1050] ("output function")
        w248 = T5 1020 items=["Single Point"=1020, "Sequence"=1021] ("source mode")
        n81 = Unbundle By Name(w232) -> ("Load channel name"=w234:string, "Load out"=w255:refnum<k15>)
        n82 = Unbundle By Name(w232) -> ("Measure record length smu"=w242:i32, "Aperture time"=w241:dbl)
        n83 = Unbundle By Name(w232) -> ("Source terminal name"=w254:string, "Measure load and scope terminal name"=w253:string)
        n84 = call <instrlib>:"niDCPower Configure Source Mode With Channels.vi"("error in (no error)"=w233, "source mode"=w248, "channel name"=w234, "instrument handle"=w255) -> ("error out"=w246:errorcluster, "instrument handle out"=w247:refnum<k15>)  [unwired: 6 in]
        n85 = call <instrlib>:"niDCPower Configure Output Function.vi"("error in (no error)"=w246, "output function"=w249, "channel name"=w234, "instrument handle"=w247) -> ("error out"=w251:errorcluster, "instrument handle out"=w250:refnum<k15>)  [unwired: 6 out]
        n86 = call-poly <instrlib>:"niDCPower Configure Trigger With Channels (Poly).vi"("error in (no error)"=w251, "input terminal"=w254, "channel name"=w234, "instrument handle"=w250) -> ("error out"=w243:errorcluster, "instrument handle out"=w252:refnum<k15>)  [unwired: 6 in]
        n87 = property class="niDCPower"(reference=w252, error in=w243, "Measure Record Length"=w242, "Aperture Time"=w241) -> (reference out=w245:refnum<k15>, error out=w244:errorcluster)
        n88 = call-poly <instrlib>:"niDCPower Configure Trigger With Channels (Poly).vi"("error in (no error)"=w244, "input terminal"=w253, "channel name"=w234, "instrument handle"=w245) -> ("error out"=w238:errorcluster, "instrument handle out"=w236:refnum<k15>)  [unwired: 6 in]
        n89 = property class="niDCPower"(reference=w236, error in=w238, "Measure When"=w239) -> (reference out=w235:refnum<k15>, error out=w237:errorcluster)
        n90 = call <instrlib>:"niDCPower Commit With Channels.vi"("error in (no error)"=w237, "channel name"=w234, "instrument handle"=w235) -> ("error out"=w230:errorcluster, "instrument handle out"=w240:refnum<k15>)  [unwired: 7 in]
        n91 = Bundle By Name(cluster=w232, "Load out"=w240) -> (w231:T3)
      }
      frame "StartSource" {
        n92 = Unbundle By Name(w261) -> ("Source out"=w257:refnum<k15>, "Source channel name"=w263:string)
        n93 = flat-sequence {
          tunnel: [w272] -> w267
          tunnel: [w271] -> w266
          tunnel: w257 -> [w270]
          tunnel: w263 -> [w268]
          tunnel: [w268] -> w265
          tunnel: w262 -> [w269]
          tunnel: w267 -> [w277]
          tunnel: w266 -> [w276]
          tunnel: [w274] -> w264
          tunnel: [w275] -> w259
          tunnel: w265 -> [w273]
          frame #0 {
            n94 = call <instrlib>:"niDCPower Initiate With Channels.vi"("error in (no error)"=w269, "channel name"=w268, "instrument handle"=w270) -> ("error out"=w271:errorcluster, "instrument handle out"=w272:refnum<k15>)  [unwired: 7 in]
          }
          frame #1 {
            w278 = T4 1033 items=["Source Complete Event"=1030, "Measure Complete Event"=1031, "Sequence Iteration Complete Event"=1032, "Sequence Engine Done Event"=1033] ("event")
            n95 = call <instrlib>:"niDCPower Wait For Event With Channels.vi"("error in (no error)"=w276, "event"=w278, "channel name"=w273, "instrument handle"=w277) -> ("error out"=w275:errorcluster, "instrument handle out"=w274:refnum<k15>)  [unwired: 6 in]
          }
        }
        n96 = Bundle By Name(cluster=w261, "Source out"=w264) -> (w260:T3)
      }
      frame "StartSourceandLoad" {
        n97 = Unbundle By Name(w281) -> ("Source out"=w283:refnum<k15>, "Source channel name"=w284:string, "Load out"=w287:refnum<k15>, "Load channel name"=w288:string)
        n98 = flat-sequence {
          tunnel: [w301] -> w292
          tunnel: [w300] -> w291
          tunnel: [w299] -> w290
          tunnel: w287 -> [w298]
          tunnel: w283 -> [w297]
          tunnel: w284 -> [w294]
          tunnel: w288 -> [w295]
          tunnel: [w294] -> w289
          tunnel: w282 -> [w296]
          tunnel: w292 -> [w308]
          tunnel: w291 -> [w307]
          tunnel: w290 -> [w304]
          tunnel: [w305] -> w285
          tunnel: [w306] -> w279
          tunnel: [w304] -> w286
          tunnel: w289 -> [w303]
          frame #0 {
            n99 = call <instrlib>:"niDCPower Initiate With Channels.vi"("error in (no error)"=w296, "channel name"=w295, "instrument handle"=w298) -> ("error out"=w302:errorcluster, "instrument handle out"=w299:refnum<k15>)  [unwired: 7 in]
            n100 = call <instrlib>:"niDCPower Initiate With Channels.vi"("error in (no error)"=w302, "channel name"=w294, "instrument handle"=w297) -> ("error out"=w300:errorcluster, "instrument handle out"=w301:refnum<k15>)  [unwired: 7 in]
          }
          frame #1 {
            w309 = T4 1033 items=["Source Complete Event"=1030, "Measure Complete Event"=1031, "Sequence Iteration Complete Event"=1032, "Sequence Engine Done Event"=1033] ("event")
            n101 = call <instrlib>:"niDCPower Wait For Event With Channels.vi"("error in (no error)"=w307, "event"=w309, "channel name"=w303, "instrument handle"=w308) -> ("error out"=w306:errorcluster, "instrument handle out"=w305:refnum<k15>)  [unwired: 6 in]
          }
        }
        n102 = Bundle By Name(cluster=w281, "Source out"=w285, "Load out"=w286) -> (w280:T3)
      }
      frame "StartSourceAndScope" {
        n103 = Unbundle By Name(w317) -> ("Source out"=w320:refnum<k15>, "Source channel name"=w319:string, "Scope out"=w315:refnum<k15>)
        n104 = flat-sequence {
          tunnel: [w331] -> w323
          tunnel: [w330] -> w322
          tunnel: w320 -> [w329]
          tunnel: w319 -> [w324]
          tunnel: [w324] -> w321
          tunnel: w316 -> [w328]
          tunnel: w315 -> [w326]
          tunnel: [w325] -> w314
          tunnel: w323 -> [w337]
          tunnel: w322 -> [w336]
          tunnel: [w334] -> w318
          tunnel: [w335] -> w313
          tunnel: w321 -> [w333]
          tunnel: [w332] -> w310
          tunnel: w314 -> [w332]
          frame #0 {
            n105 = call <instrlib>:"niScope Initiate Acquisition.vi"("instrument handle"=w326, "error in"=w328) -> ("instrument handle out"=w325:refnum<k15>, "error out"=w327:errorcluster)  [unwired: 12 in]
            n106 = call <instrlib>:"niDCPower Initiate With Channels.vi"("error in (no error)"=w327, "channel name"=w324, "instrument handle"=w329) -> ("error out"=w330:errorcluster, "instrument handle out"=w331:refnum<k15>)  [unwired: 7 in]
          }
          frame #1 {
            w338 = T4 1033 items=["Source Complete Event"=1030, "Measure Complete Event"=1031, "Sequence Iteration Complete Event"=1032, "Sequence Engine Done Event"=1033] ("event")
            n107 = call <instrlib>:"niDCPower Wait For Event With Channels.vi"("error in (no error)"=w336, "event"=w338, "channel name"=w333, "instrument handle"=w337) -> ("error out"=w335:errorcluster, "instrument handle out"=w334:refnum<k15>)  [unwired: 6 in]
          }
        }
        n108 = Bundle By Name(cluster=w317, "Source out"=w318, "Scope out"=w310) -> (w312:T3)
      }
      frame "StartSourceLoadAndScope" {
        n109 = Unbundle By Name(w341) -> ("Source out"=w350:refnum<k15>, "Source channel name"=w349:string, "Load out"=w344:refnum<k15>, "Load channel name"=w343:string, "Scope out"=w346:refnum<k15>)
        n110 = flat-sequence {
          tunnel: [w367] -> w355
          tunnel: [w366] -> w354
          tunnel: [w365] -> w353
          tunnel: w344 -> [w364]
          tunnel: w350 -> [w363]
          tunnel: w349 -> [w357]
          tunnel: w343 -> [w358]
          tunnel: [w357] -> w352
          tunnel: w342 -> [w362]
          tunnel: w346 -> [w360]
          tunnel: [w359] -> w351
          tunnel: w355 -> [w375]
          tunnel: w354 -> [w374]
          tunnel: w353 -> [w371]
          tunnel: [w372] -> w348
          tunnel: [w373] -> w339
          tunnel: [w371] -> w347
          tunnel: w352 -> [w370]
          tunnel: [w369] -> w345
          tunnel: w351 -> [w369]
          frame #0 {
            n111 = call <instrlib>:"niScope Initiate Acquisition.vi"("instrument handle"=w360, "error in"=w362) -> ("instrument handle out"=w359:refnum<k15>, "error out"=w361:errorcluster)  [unwired: 12 in]
            n112 = call <instrlib>:"niDCPower Initiate With Channels.vi"("error in (no error)"=w361, "channel name"=w358, "instrument handle"=w364) -> ("error out"=w368:errorcluster, "instrument handle out"=w365:refnum<k15>)  [unwired: 7 in]
            n113 = call <instrlib>:"niDCPower Initiate With Channels.vi"("error in (no error)"=w368, "channel name"=w357, "instrument handle"=w363) -> ("error out"=w366:errorcluster, "instrument handle out"=w367:refnum<k15>)  [unwired: 7 in]
          }
          frame #1 {
            w376 = T4 1033 items=["Source Complete Event"=1030, "Measure Complete Event"=1031, "Sequence Iteration Complete Event"=1032, "Sequence Engine Done Event"=1033] ("event")
            n114 = call <instrlib>:"niDCPower Wait For Event With Channels.vi"("error in (no error)"=w374, "event"=w376, "channel name"=w370, "instrument handle"=w375) -> ("error out"=w373:errorcluster, "instrument handle out"=w372:refnum<k15>)  [unwired: 6 in]
          }
        }
        n115 = Bundle By Name(cluster=w341, "Source out"=w348, "Load out"=w347, "Scope out"=w345) -> (w340:T3)
      }
      frame "PerformMeasurement" {
        n116 = Unbundle By Name(w392) -> ("Load enable/disable"=w419:bool, "Scope enable/disable"=w377:bool)
        n117 = Unbundle By Name(w392) -> ("Source sample rate"=w389:dbl, "Source voltatge V2 time"=w391:dbl, "Source voltage V1 time"=w390:dbl)
        n118 = Unbundle By Name(w430) -> ("Scope out"=w425:refnum<k15>, "Scope channel name"=w424:string, "Measure record length scope"=w395:i32, "measurement results.Source voltage dt"=w401:dbl)
        n119 = Unbundle By Name(w430) -> ("Source out"=w427:refnum<k15>, "Source channel name"=w426:string, "Measure record length smu"=w387:i32, "Load out"=w417:refnum<k15>, "Load channel name"=w416:string)
        n120 = Multiply(x=w389, y=w391) -> (x*y=w380:dbl)
        n121 = Multiply(x=w389, y=w390) -> (x*y=w381:dbl)
        n122 = To Long Integer(number=w381) -> (32bit integer=w378:i32)
        n123 = To Long Integer(number=w380) -> (32bit integer=w379:i32)
        n124 = Add(x=w379, y=w378) -> (x+y=w388:i32)
        n125 = Subtract(x=w387, y=w388) -> (x-y=w386:i32)
        n126 = call <instrlib>:"niDCPower Fetch Multiple.vi"("instrument handle"=w427, "channel name"=w426, "count (1)"=w387, "error in (no error)"=w431) -> ("instrument handle out"=w423:refnum<k15>, "voltage measurements"=w405:dbl[], "error out"=w420:errorcluster)  [unwired: 1 in, 8 out]
        n127 = case shown="True" w419 {
          tunnel: w420 -> [w433 w440]
          tunnel: [w433 w439] -> w418
          tunnel: w417 -> [w432 w438]
          tunnel: w416 -> [_ w437]
          tunnel: w387 -> [_ w436]
          tunnel: [w432 w435] -> w415
          tunnel: [_ w434] -> w414
          frame False {
          }
          frame True {
            n128 = call <instrlib>:"niDCPower Fetch Multiple.vi"("instrument handle"=w438, "channel name"=w437, "count (1)"=w436, "error in (no error)"=w440) -> ("instrument handle out"=w435:refnum<k15>, "voltage measurements"=w434:dbl[], "error out"=w439:errorcluster)  [unwired: 1 in, 8 out]
          }
        }
        n129 = case shown="True" w377 {
          tunnel: [w442 w449] -> w428
          tunnel: w418 -> [w442 w448]
          tunnel: w425 -> [w441 w447]
          tunnel: w424 -> [_ w446]
          tunnel: [w441 w445] -> w411
          tunnel: w395 -> [_ w444]
          tunnel: [_ w443] -> w422
          frame False {
          }
          frame True {
            n130 = call-poly <instrlib>:"niScope Fetch (poly).vi"("error in"=w448, "numSamples"=w444, "channels"=w446, "instrument handle"=w447) -> ("error out"=w449:errorcluster, "wfm"=w443:waveform(dbl), "instrument handle out"=w445:refnum<k15>)  [unwired: 4 in, 1 out]
          }
        }
        n131 = Unbundle By Name(w422) -> ("Y"=w413:dbl[], "dt"=w412:dbl)
        n132 = Unbundle By Name(w392) -> ("Source ramp stop percentage(%)"=w404:dbl, "Source ramp start percentage(%)"=w410:dbl)
        n133 = Multiply(x=w386, y=w404) -> (x*y=w408:dbl)
        n134 = Multiply(x=w386, y=w410) -> (x*y=w409:dbl)
        n135 = Divide(x=w408, y=100.0) -> (x/y=w394:dbl)
        n136 = Divide(x=w409, y=100.0) -> (x/y=w393:dbl)
        n137 = To Long Integer(number=w393) -> (32bit integer=w384:i32)
        n138 = To Long Integer(number=w394) -> (32bit integer=w385:i32)
        n139 = Add(x=w378, y=w385) -> (x+y=w382:i32)
        n140 = Add(x=w378, y=w384) -> (x+y=w383:i32)
        n141 = Index Array(array=w405, index=w382) -> (element=w403:dbl)
        n142 = Index Array(array=w405, index=w383) -> (element=w402:dbl)
        n143 = Multiply(x=w401, y=w382) -> (x*y=w400:dbl)
        n144 = Multiply(x=w401, y=w383) -> (x*y=w399:dbl)
        n145 = Subtract(x=w400, y=w399) -> (x-y=w397:dbl)
        n146 = Subtract(x=w403, y=w402) -> (x-y=w398:dbl)
        n147 = Divide(x=w398, y=w397) -> (x/y=w396:dbl)
        n148 = Bundle By Name(cluster=w430, "Source out"=w423, "measurement results.Source voltages"=w405, "Load out"=w415, "measurement results.Load voltages"=w414, "Scope out"=w411, "measurement results.Scope amplitudes"=w413, "measurement results.Scope amplitude dt"=w412, "measurement results.Ramp stop voltage level"=w403, "measurement results.Ramp start voltage level"=w402, "measurement results.Ramp stop time"=w400, "measurement results.Ramp start time"=w399, "measurement results.Actual ramp rate"=w396) -> (w429:T3)
      }
      frame "Exit", Default {
        n149 = Unbundle By Name(w462) -> ("Scope enable/disable"=w457:bool, "Load enable/disable"=w453:bool)
        n150 = Unbundle By Name(w463) -> ("Source out"=w458:refnum<k15>, "Source channel name"=w459:string, "Load out"=w451:refnum<k15>, "Load channel name"=w450:string, "Scope out"=w452:refnum<k15>)
        n151 = case shown="True" w457 {
          tunnel: w466 -> [w474 w477]
          tunnel: [w474 w476] -> w455
          tunnel: w452 -> [_ w475]
          frame False {
          }
          frame True {
            n152 = call <instrlib>:"niScope Close.vi"("instrument handle"=w475, "error in"=w477) -> ("error out"=w476:errorcluster)  [unwired: 13 in]
          }
        }
        n153 = case shown="True" w453 {
          tunnel: w455 -> [w467 w471]
          tunnel: [w467 w470] -> w454
          tunnel: w451 -> [_ w469]
          tunnel: w450 -> [_ w468]
          frame False {
          }
          frame True {
            n154 = call <instrlib>:"niDCPower Abort With Channels.vi"("error in (no error)"=w471, "channel name"=w468, "instrument handle"=w469) -> ("error out"=w473:errorcluster, "instrument handle out"=w472:refnum<k15>)  [unwired: 7 in]
            n155 = call <instrlib>:"niDCPower Close.vi"("error in (no error)"=w473, "instrument handle"=w472) -> ("error out"=w470:errorcluster)  [unwired: 9 in]
          }
        }
        n156 = call <instrlib>:"niDCPower Abort With Channels.vi"("error in (no error)"=w454, "channel name"=w459, "instrument handle"=w458) -> ("error out"=w461:errorcluster, "instrument handle out"=w460:refnum<k15>)  [unwired: 7 in]
        n157 = call <instrlib>:"niDCPower Close.vi"("error in (no error)"=w461, "instrument handle"=w460) -> ("error out"=w465:errorcluster)  [unwired: 9 in]
      }
    }
  }
  "error out" <- w8
  "measure call context out" <- w1
  n158 = Unbundle By Name(w6) -> ("measurement results"=→"measurement results":T2)
